vi "Expow.vi"(0 "Expo1[ms]":i32[](array[numeric]), 1 "Numeric":i32) -> ()   [LabVIEW 2014]
uses:
  wlmData.dll
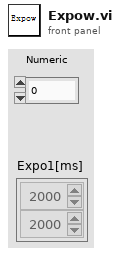
[diagram p1: front panel]
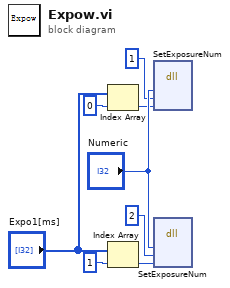
[diagram p0: block diagram]
diagram:
  n1 = Index Array(array="Expo1[ms]", index=0) -> (element=w2:i32)
  n2 = Index Array(array="Expo1[ms]", index=1) -> (element=w1:i32)
  n3 = dll-call lib="wlmData.dll" fn="SetExposureNum"("num"="Numeric", "arr"=1, "E"=w2) -> ()  [unwired: 7 in, 2 out]
  n4 = dll-call lib="wlmData.dll" fn="SetExposureNum"("num"="Numeric", "arr"=2, "E"=w1) -> ()  [unwired: 7 in, 2 out]
